vi "Destruct Messenger.vi"(8 "error in (no error)":errorcluster, 11 "Messenger Composite Component in":refnum<class "Messenger Composite.lvclass">) -> (0 "error out":errorcluster, 3 "Messenger Composite Component out":refnum<class "Messenger Composite.lvclass">)   [LabVIEW 2024, in "Messenger Composite.lvclass"]
uses:
  Messenger Composite.lvclass
  Messenger Composite.lvclass/Messenger Composite.ctl
  Messenger/Messenger.lvclass
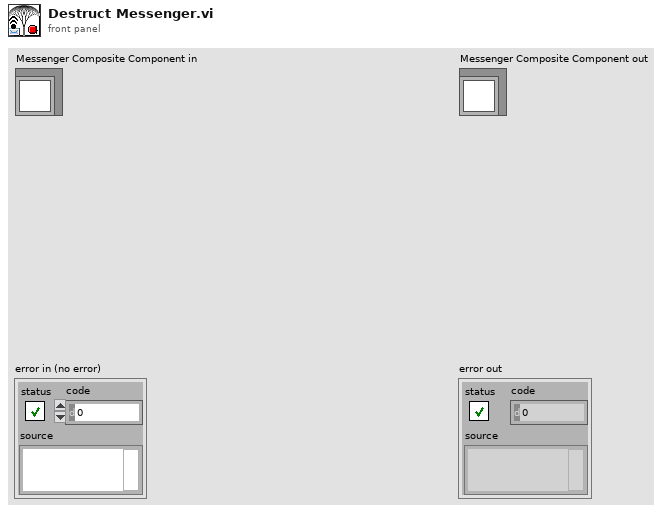
[diagram p1: front panel]
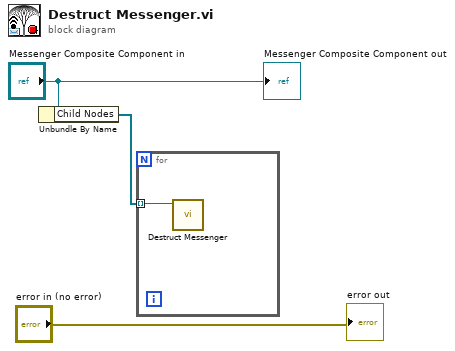
[diagram p0: block diagram]
diagram:
  n1 = Unbundle By Name("Messenger Composite Component in") -> ("Child Nodes"=w2:refnum<class "Messenger.lvclass">[])
  n2 = for {
    tunnel: w2 -> [w4] mode=indexing
    n3 = call-dynamic "Destruct Messenger.vi"("Messenger Component in"=w4) -> ()  [unwired: 9 in, 2 out]
  }
  "error out" <- "error in (no error)"
  "Messenger Composite Component out" <- "Messenger Composite Component in"
